vi "Tests.vi"(8 "error in (no error)":errorcluster) -> (0 "error out":errorcluster)   [LabVIEW 2019]
uses:
  <vilib>/addons/_JKI Toolkits/Caraya/classes/Test/Test.lvclass
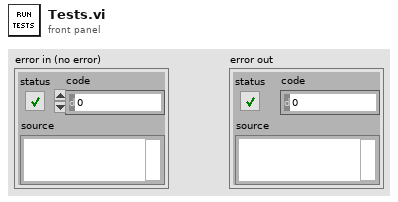
[diagram p1: front panel]
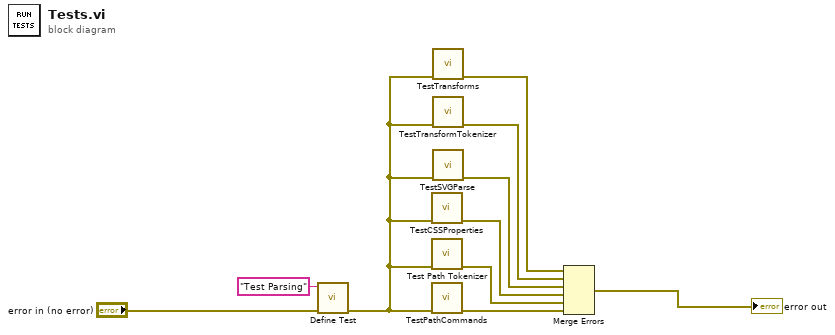
[diagram p0: block diagram]
diagram:
  n1 = call <vilib>:"Define Test.vi"("error in (no error)"="error in (no error)", "Label (VI Title)"="Test Parsing") -> ("error out"=w6:errorcluster)  [unwired: 8 in, 1 out]
  n2 = call "TestCSSProperties.vi"("error in (no error)"=w6) -> ("error out"=w4:errorcluster)  [unwired: 10 in]
  n3 = call "Test Path Tokenizer.vi"("error in (no error)"=w6) -> ("error out"=w5:errorcluster)  [unwired: 10 in]
  n4 = call "TestPathCommands.vi"("error in (no error)"=w6) -> ("error out"=w10:errorcluster)  [unwired: 10 in]
  n5 = call "TestTransforms.vi"("error in (no error)"=w6) -> ("error out"=w1:errorcluster)  [unwired: 10 in]
  n6 = call "TestTransformTokenizer.vi"("error in (no error)"=w6) -> ("error out"=w2:errorcluster)  [unwired: 10 in]
  n7 = call "TestSVGParse.vi"("error in (no error)"=w6) -> ("error out"=w3:errorcluster)  [unwired: 10 in]
  n8 = Merge Errors(w1, w2, w3, w4, w5, w10) -> (→"error out":errorcluster)
